vi "Actor Core.vi"(8 "error in":errorcluster, 11 "Form Window in":refnum<class "Form Window.lvclass">) -> (0 "error out":errorcluster, 3 "Actor out":refnum<class "Actor.lvclass">)   [LabVIEW 2020, in "Panel Form Controller.lvlib" / "Form Window.lvclass"]
doc: "The user interface for this panel.\n\n----\nPlease see the following web address for additional documentation and tutorial information:\nhttp://www.mooregoodideas.com/mgi-panel-manager/\n\nAuthor: Derek Trepanier\n\nCopyright (c) 2018, Moore Good Ideas, Inc.\n\nAll rights reserved.\n\nRedistribution and use in source and binary forms, with or without modification, are permitted provided that the following conditions are met:\n\n * Redistributions of source code must retain the above copyright notice, this list of conditions and the following disclaimer.\n * Redistributions in binary form must reproduce the above copyright notice, this list of conditions and the following disclaimer in the documentation and/or other materials provided with the distribution.\n * Neither the name of Moore Good Ideas, Inc. nor the names of its contributors may be used to endorse or promote products derived from this software without specific prior written permission.\n\nTHIS SOFTWARE IS PROVIDED BY THE COPYRIGHT HOLDERS AND CONTRIBUTORS \"AS IS\" AND ANY EXPRESS OR IMPLIED WARRANTIES, INCLUDING, BUT NOT LIMITED TO, THE IMPLIED WARRANTIES OF MERCHANTABILITY AND FITNESS FOR A PARTICULAR PURPOSE ARE DISCLAIMED. IN NO EVENT SHALL THE COPYRIGHT OWNER OR CONTRIBUTORS BE LIABLE FOR ANY DIRECT, INDIRECT, INCIDENTAL, SPECIAL, EXEMPLARY, OR CONSEQUENTIAL DAMAGES (INCLUDING, BUT NOT LIMITED TO, PROCUREMENT OF SUBSTITUTE GOODS OR SERVICES; LOSS OF USE, DATA, OR PROFITS; OR BUSINESS INTERRUPTION) HOWEVER CAUSED AND ON ANY THEORY OF LIABILITY, WHETHER IN CONTRACT, STRICT LIABILITY, OR TORT (INCLUDING NEGLIGENCE OR OTHERWISE) ARISING IN ANY WAY OUT OF THE USE OF THIS SOFTWARE, EVEN IF ADVISED OF THE POSSIBILITY OF SUCH DAMAGE."
uses:
  Form Window.lvclass
  C:/Users/User/Desktop/Raman Program/LV-Database-OOP/source/Forms AF/Forms Controller/Form Controller/Panel Form Controller.lvclass
  C:/Program Files (x86)/National Instruments/LabVIEW 2020/vi.lib/ActorFramework/Actor/Actor.lvclass
  <vilib>/ActorFramework/Actor/Actor.lvclass
  Form Controller/Panel Form Controller.lvclass/Panel Form Controller.ctl
  Configuration/Controller Configuration/Panel Form Controller Configuration.lvclass/Panel Form Controller Configuration.ctl
  Add Row to Database/Add Row to Database.lvclass
  C:/Users/User/Desktop/Raman Program/LV-Database-OOP/source/Database OOP/Button Libraries/Button Interface Class/Button Interface.lvclass
  <vilib>/ActorFramework/Actor/Actor.lvclass/Actor.ctl
  <vilib>/ActorFramework/Message Enqueuer/Message Enqueuer.lvclass/Message Enqueuer.ctl
  <vilib>/ActorFramework/Message Enqueuer/Init from Existing Queue.vi
  Configuration/Controller Configuration/Panel Form Controller Configuration.lvclass
  <vilib>/ActorFramework/Message Enqueuer/Message Enqueuer.lvclass
  Database OOP/Table Libraries/Basic Form/Basic Form.lvclass
  Form Controller/Panel Form Controller.lvclass
panel:
  in  "Add":bool
  in  "Primary Key":u16(ring)
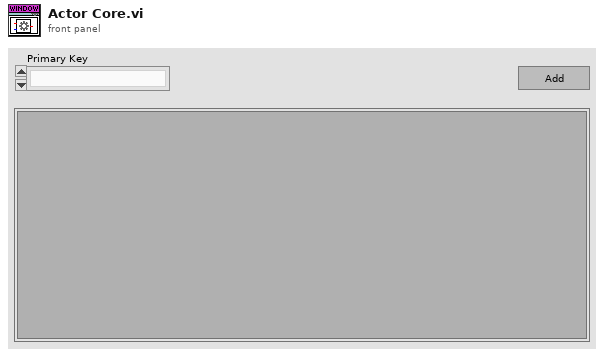
[diagram p1: front panel]
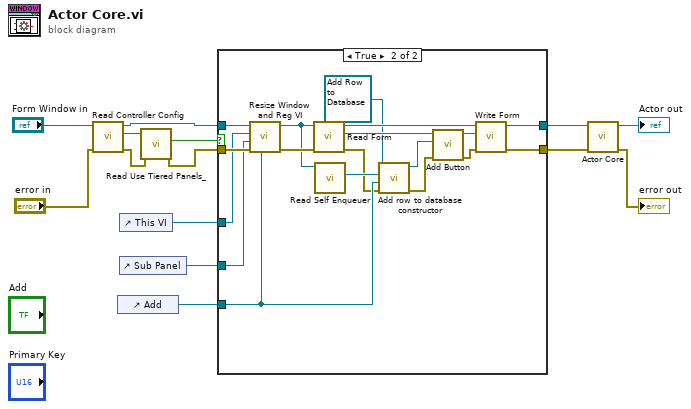
[diagram p0: block diagram]
diagram:
  n1 = call "Read Controller Config.vi"("error in (no error)"="error in", "Panel Form Controller in"="Form Window in") -> ("error out"=w11:errorcluster, "Controller Config"=w12:refnum<class "Panel Form Controller Configuration.lvclass">, "Panel Form Controller out"=w9:refnum<class "Form Window.lvclass">)  [unwired: 7 in]
  n2 = control-ref of="Add"() -> (w5:refnum<vi>)
  n3 = control-ref of="This VI"() -> (w7:refnum<vi>)
  n4 = control-ref of="Sub Panel"() -> (w6:refnum<vi>)
  n5 = call "Read Use Tiered Panels_.vi"("error in (no error)"=w11, "Panel Form Controller Configuration in"=w12) -> ("error out"=w8:errorcluster, "Use Tiered Panels?"=w10:bool)  [unwired: 7 in, 1 out]
  n6 = case shown="True" w10 {
    tunnel: [w16 w29] -> w4
    tunnel: [w15 w27] -> w3
    tunnel: w9 -> [w16 w30]
    tunnel: w8 -> [w15 w34]
    tunnel: w7 -> [_ w31]
    tunnel: w6 -> [_ w32]
    tunnel: w5 -> [_ w21]
    frame False {
    }
    frame True {
      n7 = call "Resize Window and Reg VI.vi"("Add Button Refnum"=w21, "error in (no error)"=w34, "Sub Panel Refnum"=w32, "Actor Core Refnum"=w31, "Form Window in"=w30) -> ("error out"=w33:errorcluster, "Form Window out"=w23:refnum<class "Form Window.lvclass">)  [unwired: 5 in]
      n8 = call "Read Form.vi"("error in (no error)"=w33, "Panel Form Controller in"=w23) -> ("error out"=w20:errorcluster, "Form"=w25:refnum<class "Basic Form.lvclass">, "Panel Form Controller out"=w28:refnum<class "Form Window.lvclass">)  [unwired: 7 in]
      n9 = call <vilib>:"Read Self Enqueuer.vi"("Actor"=w23) -> ("Self Enqueuer"=w22:refnum<class "Message Enqueuer.lvclass">)  [unwired: 10 in]
      n10 = call "Add row to database constructor.vi"("error in (no error)"=w20, "Ctl Refnum"=w21, "Self Enqueuer"=w22, "Add Row to Database in"=refnum<class "Add Row to Database.lvclass"> refnum) -> ("error out"=w19:errorcluster, "Add Row to Database out"=w26:refnum<class "Add Row to Database.lvclass">)  [unwired: 6 in]
      n11 = call "Add Button.vi"("error in (no error)"=w19, "Button"=w26, "Basic Form in"=w25) -> ("error out"=w18:errorcluster, "Basic Form out"=w24:refnum<class "Basic Form.lvclass">)  [unwired: 7 in]
      n12 = call "Write Form.vi"("error in (no error)"=w18, "Form.lvlib:Basic Form.lvclass"=w24, "Panel Form Controller in"=w28) -> ("error out"=w27:errorcluster, "Panel Form Controller out"=w29:refnum<class "Form Window.lvclass">)  [unwired: 7 in]
    }
  }
  n13 = call-parent "Actor Core.vi"("error in"=w3, "Panel Form Controller in"=w4) -> ("error out"=→"error out":errorcluster, "Actor out"=→"Actor out":refnum<class "Actor.lvclass">)  [unwired: 8 in]
